vi "log in.vi"() -> ()   [LabVIEW 2016]
uses:
  <vilib>/Utility/config.llb/Read Key (Boolean).vi
  <vilib>/Utility/config.llb/Write Key (String).vi
  <vilib>/Utility/config.llb/Write Key (Boolean).vi
  <vilib>/Utility/config.llb/Read Key (String).vi
  <vilib>/smtpClient/Set Message Text.vi
  <vilib>/Utility/config.llb/NI_LVConfig.lvlib
  <vilib>/smtpClient/LabVIEWSMTPClient.lvlib
panel:
  in  "Sair":bool
  out "error out":errorcluster
  in  "nagevação":enum32{"log in", "cadastrar novo usuário"}(tab)
  in  "Esqueceu a senha":bool
  out "errada":string="Senha ou Usuários incorretos"
  in  "Senha":string
  in  "Usuário":string
  in  "Entrar":bool
  in  "remember":bool
  in  "novo_user":bool
  in  "Voltar":bool
  in  "novamente":string caption="Digite a senha novamente"
  in  "Digite a senha":string
  in  "Usuário":string
  in  "Cadastrar":bool
  # "Cadastrar novo usuário"
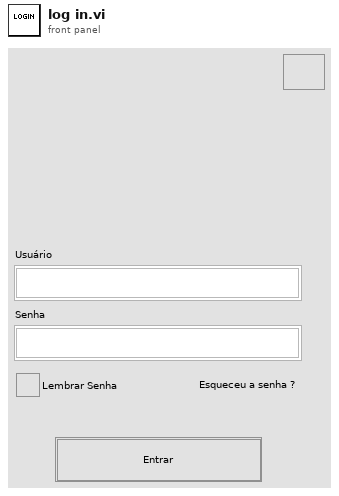
[diagram p1: front panel]
types:
  T1 = typedef "NI_LVConfig.lvlib/Config Data RefNum.ctl" = refnum<k1>
  T2 = typedef "LabVIEWSMTPClient.lvlib/SmtpClientHandle.ctl" = refnum<k1>
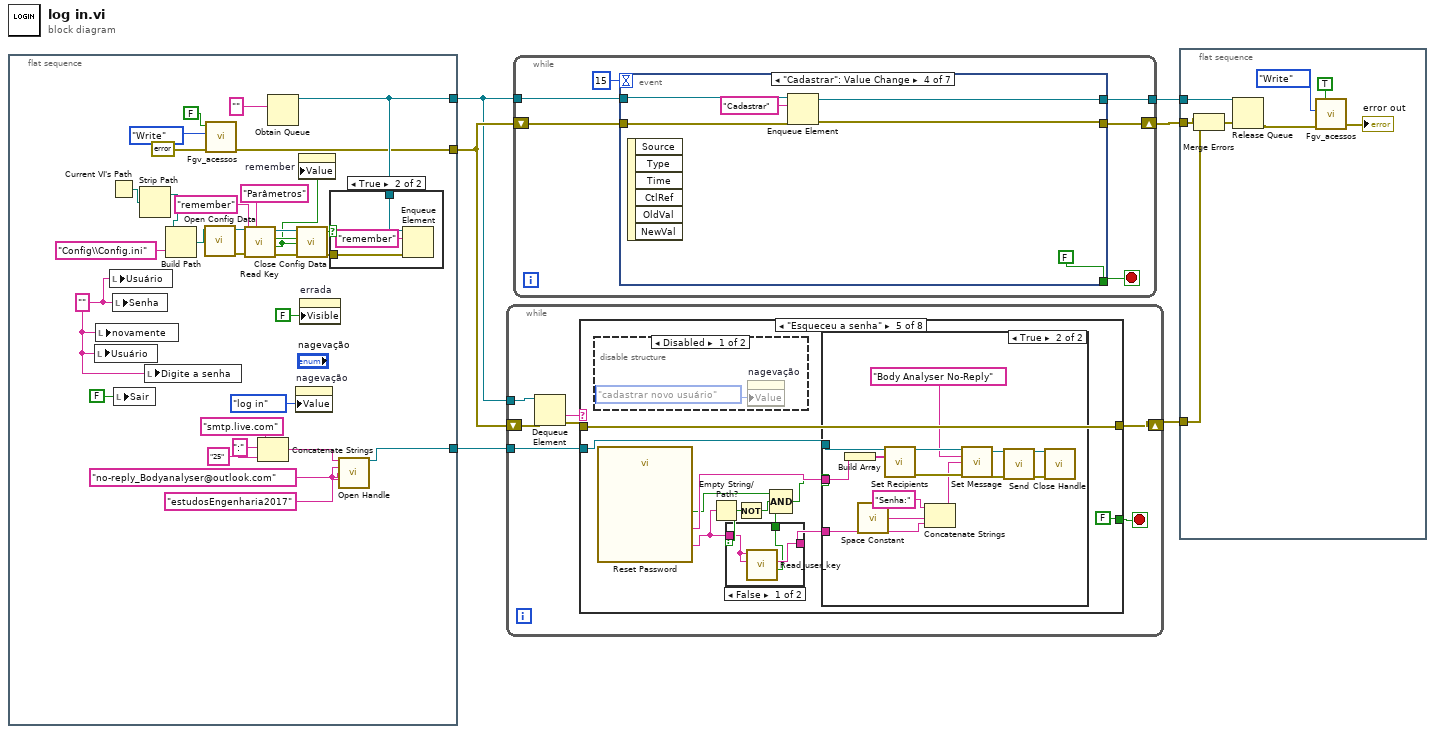
[diagram p0: block diagram]
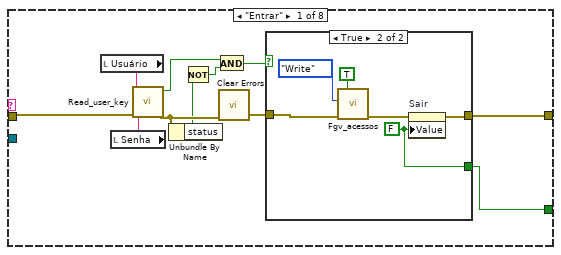
[diagram p2: hidden frame]
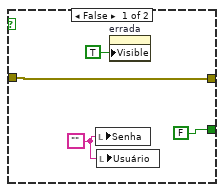
[diagram p3: hidden frame]
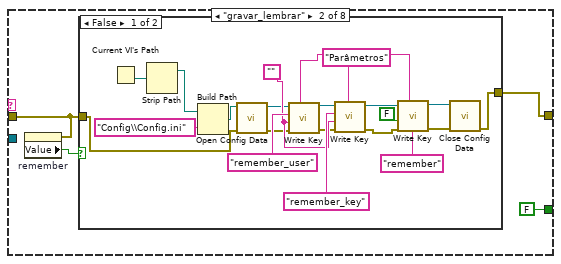
[diagram p4: hidden frame]
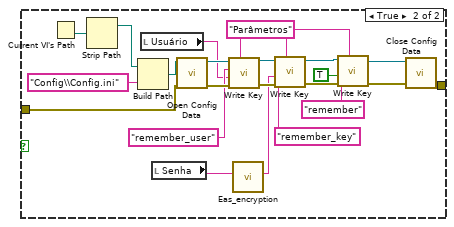
[diagram p5: hidden frame]
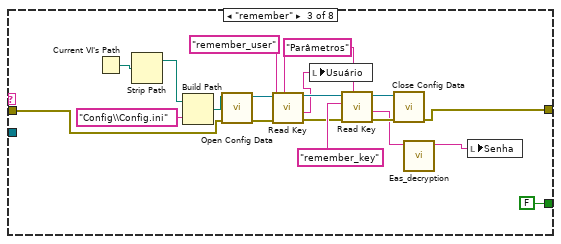
[diagram p6: hidden frame]
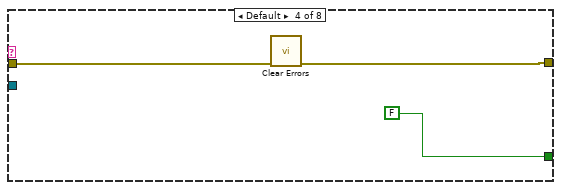
[diagram p7: hidden frame]
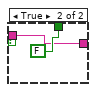
[diagram p8: hidden frame]
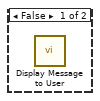
[diagram p9: hidden frame]
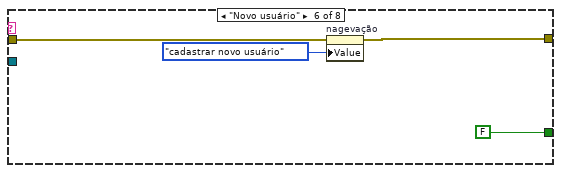
[diagram p11: hidden frame]
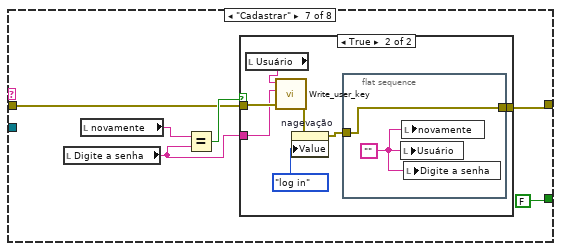
[diagram p12: hidden frame]
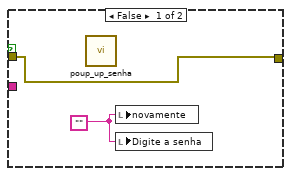
[diagram p13: hidden frame]
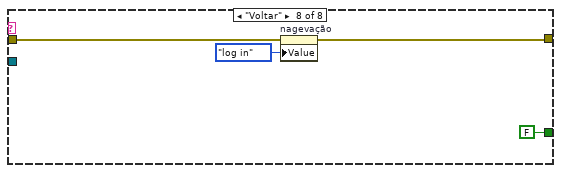
[diagram p14: hidden frame]
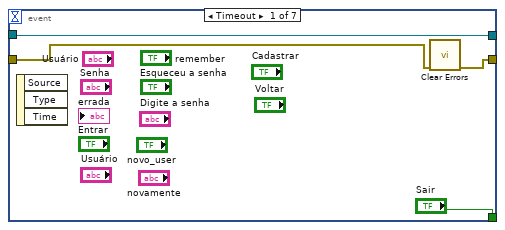
[diagram p15: hidden frame]
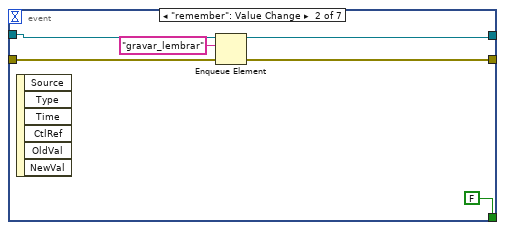
[diagram p16: hidden frame]
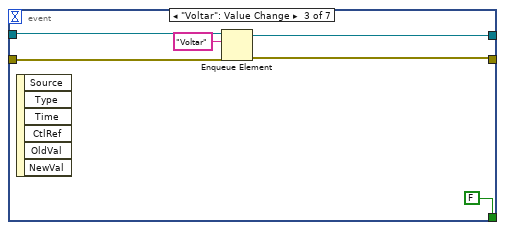
[diagram p17: hidden frame]
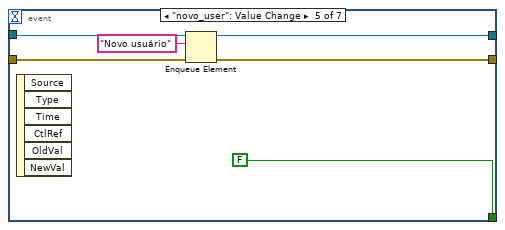
[diagram p18: hidden frame]
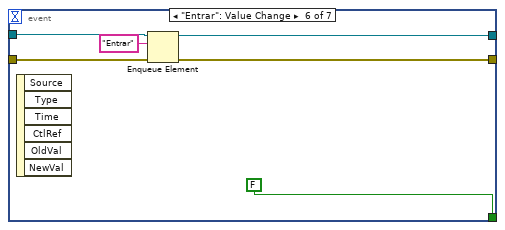
[diagram p19: hidden frame]
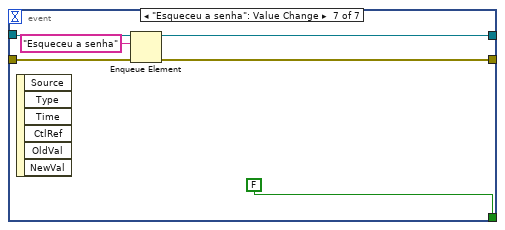
[diagram p20: hidden frame]
diagram:
  n1 = flat-sequence {
    tunnel: [w16] -> w6
    tunnel: [w17] -> w3
    tunnel: [w7] -> w1
    frame #0 {
      w9 = "no-reply_Bodyanalyser@outlook.com" ("from")
      w32 = "" ("Senha")
      n2 = local write "Usuário"(w32) -> ()
      n3 = local write "novamente"(w32) -> ()
      n4 = Current VI's Path() -> (path=w23:path)
      n5 = local write "Usuário"(w32) -> ()
      n6 = local write "Senha"(w32) -> ()
      n7 = local write "Sair"(FALSE ("Sair")) -> ()
      n8 = Strip Path(path=w23) -> (stripped path=w22:path)  [unwired: 1 out]
      n9 = local write "Digite a senha"(w32) -> ()
      n10 = Build Path(base path=w22, name or relative path="Config\\Config.ini") -> (appended path=w20:path)
      n11 = call <vilib>:"Open Config Data.vi"("configuration file path"=w20) -> ("error out"=w28:errorcluster, "refnum"=w27:T1)  [unwired: 8 in, 1 out]
      n12 = call "Fgv_acessos.vi"("error in"=errorcluster {"status"=FALSE, "code"=0, "source"=""} ("error constant"), "Tipo"=enum16{"Write", "Read"}."Write", "Log in _acesso"=FALSE) -> ("Error out"=w16:errorcluster)  [unwired: 7 in, 1 out]
      n13 = call-poly <vilib>:"Read Key.vi"("section"="Parâmetros", "error in (no error)"=w28, "key"="remember", "refnum"=w27) -> ("error out"=w26:errorcluster, "value"=w14:bool, "found?"=w25:bool, "refnum out"=w24:T1)  [unwired: 4 in]
      n14 = Concatenate Strings("smtp.live.com" ("server address"), ":" ("string"), "25" ("string")) -> (w10:string)
      n15 = Obtain Queue(element data type="" ("name (unnamed)")) -> (queue out=w17:refnum<queue>)  [unwired: 4 in, 2 out]
      n16 = property on="nagevação" class="TabCtl (strict)"("Value"=enum32{"log in", "cadastrar novo usuário"}."log in" ("nagevação")) -> ()  [unwired: 2 in, 2 out]
      n17 = call <vilib>:"Close Config Data.vi"("error in (no error)"=w26, "write file if changed (T)"=w25, "refnum"=w24) -> ("error out"=w15:errorcluster)  [unwired: 7 in, 1 out]
      n18 = property on="remember" class="Bool (strict)"("Value"=w14) -> ()  [unwired: 2 in, 2 out]
      n19 = property on="errada" class="Str"("Visible"=FALSE) -> ()  [unwired: 2 in, 2 out]
      n20 = case shown="True" w14 {
        tunnel: w17 -> [_ w39]
        tunnel: w15 -> [_ w38]
        frame False {
        }
        frame True {
          n21 = Enqueue Element(queue=w39, element="remember", error in (no error)=w38) -> ()  [unwired: 1 in, 3 out]
        }
      }
      n22 = call <vilib>:"Open Handle.vi"("server address"=w10, "from"=w9, "username"=w9, "password"="estudosEngenharia2017") -> ("handle out"=w7:T2)  [unwired: 10 in, 1 out]
    }
  }
  n23 = while {
    shift-right: [w44] -> w4
    shift-left: w6 -> [w45]
    tunnel: w3 -> [w42]
    tunnel: w1 -> [w40]
    stop <- w41 stop-if-true
    n24 = Dequeue Element(queue=w42, error in (no error)=w45) -> (element=w46:string, error out=w43:errorcluster)  [unwired: 1 in, 2 out]
    n25 = case shown="\"Esqueceu a senha\"" w46 {
      tunnel: [w53 w70 w118 w133 w146 w169 w172 w189] -> w44
      tunnel: w43 -> [w57 w69 w128 w134 w146 w170 w173 w190]
      tunnel: [w54 FALSE ("Sair") FALSE ("Sair") FALSE FALSE FALSE FALSE FALSE ("Sair")] -> w41
      tunnel: w40 -> [_ _ _ _ w144 _ _ _]
      frame "Entrar" {
        n26 = local read "Usuário"() -> (w56:string)
        n27 = local read "Senha"() -> (w55:string)
        n28 = call "Read_user_key.vi"("Error in"=w57, "Senha"=w55, "User"=w56) -> ("Error out"=w51:errorcluster, "Dados Válidos"=w48:bool)  [unwired: 5 in, 2 out]
        n29 = Unbundle By Name(w51) -> ("status"=w50:bool)
        n30 = Not(x=w50) -> (.not. x?=w49:bool)
        n31 = And(x=w48, y=w49) -> (x .and. y?=w47:bool)
        n32 = call <vilib>:"Clear Errors.vi"("error in (no error)"=w51) -> ("error out"=w52:errorcluster)  [unwired: 5 in, 1 out]
        n33 = case shown="True" w47 {
          tunnel: [FALSE w67] -> w54
          tunnel: w52 -> [w58 w63]
          tunnel: [w58 w66] -> w53
          frame False {
            w60 = ""
            n34 = local write "Senha"(w60) -> ()
            n35 = local write "Usuário"(w60) -> ()
            n36 = property on="errada" class="Str"("Visible"=TRUE) -> ()  [unwired: 2 in, 2 out]
          }
          frame True {
            w67 = FALSE ("Sair")
            n37 = call "Fgv_acessos.vi"("error in"=w63, "Tipo"=enum16{"Write", "Read"}."Write", "Log in _acesso"=TRUE) -> ("Error out"=w62:errorcluster)  [unwired: 7 in, 1 out]
            n38 = property on="Sair" class="Bool (strict)"(error in=w62, "Value"=w67) -> (error out=w66:errorcluster)  [unwired: 1 in, 1 out]
          }
        }
      }
      frame "gravar_lembrar" {
        n39 = property on="remember" class="Bool (strict)"(error in=w69) -> ("Value"=w68:bool)  [unwired: 1 in, 2 out]
        n40 = case shown="False" w68 {
          tunnel: w69 -> [w87 w111]
          tunnel: [w78 w104] -> w70
          frame False {
            w76 = ""
            w86 = "Parâmetros" ("section")
            n41 = Current VI's Path() -> (path=w91:path)
            n42 = Strip Path(path=w91) -> (stripped path=w90:path)  [unwired: 1 out]
            n43 = Build Path(base path=w90, name or relative path="Config\\Config.ini") -> (appended path=w88:path)
            n44 = call <vilib>:"Open Config Data.vi"("error in (no error)"=w87, "configuration file path"=w88) -> ("error out"=w74:errorcluster, "refnum"=w75:T1)  [unwired: 7 in, 1 out]
            n45 = call-poly <vilib>:"Write Key.vi"("section"=w86, "error in (no error)"=w74, "value"=w76, "key"="remember_user", "refnum"=w75) -> ("error out"=w73:errorcluster, "refnum out"=w72:T1)  [unwired: 4 in, 1 out]
            n46 = call-poly <vilib>:"Write Key.vi"("section"=w86, "error in (no error)"=w73, "value"=w76, "key"="remember_key", "refnum"=w72) -> ("error out"=w82:errorcluster, "refnum out"=w81:T1)  [unwired: 4 in, 1 out]
            n47 = call-poly <vilib>:"Write Key.vi"("section"=w86, "error in (no error)"=w82, "value"=FALSE, "key"="remember", "refnum"=w81) -> ("error out"=w79:errorcluster, "refnum out"=w80:T1)  [unwired: 4 in, 1 out]
            n48 = call <vilib>:"Close Config Data.vi"("error in (no error)"=w79, "refnum"=w80) -> ("error out"=w78:errorcluster)  [unwired: 8 in, 1 out]
          }
          frame True {
            w96 = "Parâmetros" ("section")
            n49 = Current VI's Path() -> (path=w113:path)
            n50 = Strip Path(path=w113) -> (stripped path=w112:path)  [unwired: 1 out]
            n51 = Build Path(base path=w112, name or relative path="Config\\Config.ini") -> (appended path=w109:path)
            n52 = local read "Usuário"() -> (w101:string)
            n53 = local read "Senha"() -> (w100:string)
            n54 = call <vilib>:"Open Config Data.vi"("error in (no error)"=w111, "configuration file path"=w109) -> ("error out"=w108:errorcluster, "refnum"=w107:T1)  [unwired: 7 in, 1 out]
            n55 = call-poly <vilib>:"Write Key.vi"("section"=w96, "error in (no error)"=w108, "value"=w101, "key"="remember_user", "refnum"=w107) -> ("error out"=w106:errorcluster, "refnum out"=w105:T1)  [unwired: 4 in, 1 out]
            n56 = call "Eas_encryption.vi"("Key"=w100) -> ("Key"=w99:string)  [unwired: 8 in, 2 out]
            n57 = call-poly <vilib>:"Write Key.vi"("section"=w96, "error in (no error)"=w106, "value"=w99, "key"="remember_key", "refnum"=w105) -> ("error out"=w98:errorcluster, "refnum out"=w97:T1)  [unwired: 4 in, 1 out]
            n58 = call-poly <vilib>:"Write Key.vi"("section"=w96, "error in (no error)"=w98, "value"=TRUE, "key"="remember", "refnum"=w97) -> ("error out"=w93:errorcluster, "refnum out"=w92:T1)  [unwired: 4 in, 1 out]
            n59 = call <vilib>:"Close Config Data.vi"("error in (no error)"=w93, "refnum"=w92) -> ("error out"=w104:errorcluster)  [unwired: 8 in, 1 out]
          }
        }
      }
      frame "remember" {
        w125 = "Parâmetros" ("section")
        n60 = Current VI's Path() -> (path=w132:path)
        n61 = Strip Path(path=w132) -> (stripped path=w131:path)  [unwired: 1 out]
        n62 = Build Path(base path=w131, name or relative path="Config\\Config.ini") -> (appended path=w129:path)
        n63 = call <vilib>:"Open Config Data.vi"("error in (no error)"=w128, "configuration file path"=w129) -> ("error out"=w127:errorcluster, "refnum"=w126:T1)  [unwired: 7 in, 1 out]
        n64 = call-poly <vilib>:"Read Key.vi"("section"=w125, "error in (no error)"=w127, "key"="remember_user", "refnum"=w126) -> ("error out"=w119:errorcluster, "value"=w116:string, "refnum out"=w124:T1)  [unwired: 4 in, 1 out]
        n65 = local write "Usuário"(w116) -> ()
        n66 = call-poly <vilib>:"Read Key.vi"("section"=w125, "error in (no error)"=w119, "key"="remember_key", "refnum"=w124) -> ("error out"=w120:errorcluster, "value"=w115:string, "refnum out"=w121:T1)  [unwired: 4 in, 1 out]
        n67 = call <vilib>:"Close Config Data.vi"("error in (no error)"=w120, "refnum"=w121) -> ("error out"=w118:errorcluster)  [unwired: 8 in, 1 out]
        n68 = call "Eas_decryption.vi"("Key"=w115) -> ("Key"=w114:string)  [unwired: 9 in, 1 out]
        n69 = local write "Senha"(w114) -> ()
      }
      frame Default {
        n70 = call <vilib>:"Clear Errors.vi"("error in (no error)"=w134) -> ("error out"=w133:errorcluster)  [unwired: 5 in, 1 out]
      }
      frame "Esqueceu a senha" {
        n71 = disable-structure shown="Disabled" {
          frame Disabled {
            n72 = property on="nagevação" class="TabCtl (strict)"("Value"=enum32{"log in", "cadastrar novo usuário"}."cadastrar novo usuário" ("nagevação")) -> ()  [unwired: 2 in, 2 out]
          }
          frame Enabled {
          }
        }
        n73 = call "Reset Password"() -> ("Úsuário"=w137:string, "E-mail"=w143:string, "OK"=w141:bool)  [unwired: 16 in, 1 out]
        n74 = Empty String/Path?(string/path=w137) -> (empty?=w136:bool)
        n75 = case shown="False" w136 {
          tunnel: [w149 w150] -> w142
          tunnel: [w148 FALSE] -> w139
          tunnel: w137 -> [w147 w150]
          frame False {
            n76 = call "Read_user_key.vi"("Senha"=w147, "User"=w147) -> ("x = y?"=w148:bool, "Key"=w149:string)  [unwired: 6 in, 2 out]
          }
          frame True {
          }
        }
        n77 = Not(x=w136) -> (.not. x?=w140:bool)
        n78 = Compound Arithmetic op=AND(w141, w140, w139) -> (w138:bool)
        n79 = case shown="True" w138 {
          tunnel: w144 -> [_ w161]
          tunnel: w143 -> [_ w160]
          tunnel: w142 -> [_ w156]
          frame False {
            n80 = call "Display Message to User"() -> ()  [unwired: 10 in, 2 out]
          }
          frame True {
            n81 = Build Array(w160) -> (w159:string[])
            n82 = call <vilib>:"Space Constant.vi"() -> ("String"=w155:string)
            n83 = call <vilib>:"Set Recipients.vi"("handle in"=w161, "to"=w159) -> ("handle out"=w165:T2, "error out"=w164:errorcluster)  [unwired: 12 in]
            n84 = Concatenate Strings("Senha:" ("plain text message"), w155, w156) -> (w154:string)
            n85 = call-poly <vilib>:"Set Message.vi"("handle in"=w165, "subject"="Body Analyser No-Reply", "plain text message"=w154, "error in (no error)"=w164) -> ("handle out"=w162:T2, "error out"=w163:errorcluster)  [unwired: 10 in]
            n86 = call <vilib>:"Send.vi"("handle in"=w162, "error in (no error)"=w163) -> ("handle out"=w152:T2, "error out"=w153:errorcluster)  [unwired: 11 in, 1 out]
            n87 = call <vilib>:"Close Handle.vi"("handle in"=w152, "error in (no error)"=w153) -> ()  [unwired: 12 in, 2 out]
          }
        }
      }
      frame "Novo usuário" {
        n88 = property on="nagevação" class="TabCtl (strict)"(error in=w170, "Value"=enum32{"log in", "cadastrar novo usuário"}."cadastrar novo usuário" ("nagevação")) -> (error out=w169:errorcluster)  [unwired: 1 in, 1 out]
      }
      frame "Cadastrar" {
        n89 = local read "Digite a senha"() -> (w171:string)
        n90 = local read "novamente"() -> (w175:string)
        n91 = Equal?(x=w175, y=w171) -> (x = y?=w174:bool)
        n92 = case shown="True" w174 {
          tunnel: w173 -> [w178 w185]
          tunnel: [w178 w179] -> w172
          tunnel: w171 -> [_ w183]
          frame False {
            w177 = ""
            n93 = call "poup_up_senha.vi"() -> ()  [unwired: 12 in]
            n94 = local write "novamente"(w177) -> ()
            n95 = local write "Digite a senha"(w177) -> ()
          }
          frame True {
            n96 = local read "Usuário"() -> (w184:string)
            n97 = call "Write_user_key.vi"("Error in"=w185, "Key"=w183, "User"=w184) -> ("error out"=w181:errorcluster)  [unwired: 8 in]
            n98 = property on="nagevação" class="TabCtl (strict)"(error in=w181, "Value"=enum32{"log in", "cadastrar novo usuário"}."log in" ("nagevação")) -> (error out=w180:errorcluster)  [unwired: 1 in, 1 out]
            n99 = flat-sequence {
              tunnel: w180 -> [w187]
              tunnel: [w187] -> w179
              frame #0 {
                w186 = ""
                n100 = local write "Usuário"(w186) -> ()
                n101 = local write "novamente"(w186) -> ()
                n102 = local write "Digite a senha"(w186) -> ()
              }
            }
          }
        }
      }
      frame "Voltar" {
        n103 = property on="nagevação" class="TabCtl (strict)"(error in=w190, "Value"=enum32{"log in", "cadastrar novo usuário"}."log in" ("nagevação")) -> (error out=w189:errorcluster)  [unwired: 1 in, 1 out]
      }
    }
  }
  n104 = while {
    tunnel: w3 -> [w197]
    shift-right: [w195] -> w5
    shift-left: w6 -> [w196]
    tunnel: [w194] -> w2
    stop <- w192 stop-if-true
    n105 = event shown="[3] \"Cadastrar\": Value Change" {
      selector: _ -> [_ _ _ _ _ _ _]
      dyn-events: _ -> [_ _ _ _ _ _ _]
      timeout: 15 -> [_ _ _ _ _ _ _]
      tunnel: w197 -> [w201 w206 w213 w219 w225 w231 w237]
      tunnel: w196 -> [w198 w207 w212 w218 w224 w229 w236]
      tunnel: [w199 w204 w211 w217 w223 w228 w235] -> w195
      tunnel: [w201 w205 w210 w216 w222 w227 w233] -> w194
      tunnel: ["Sair" FALSE ("Sair") FALSE ("Sair") FALSE FALSE FALSE FALSE] -> w192
      event Timeout {
        n106 = event-data() -> ()  [unwired: 1 in, 3 out]
        n107 = call <vilib>:"Clear Errors.vi"("error in (no error)"=w198) -> ("error out"=w199:errorcluster)  [unwired: 5 in, 1 out]
      }
      event "remember": Value Change {
        n108 = event-data() -> ()  [unwired: 1 in, 6 out]
        n109 = Enqueue Element(queue=w206, element="gravar_lembrar", error in (no error)=w207) -> (queue out=w205:refnum<queue>, error out=w204:errorcluster)  [unwired: 1 in, 1 out]
      }
      event "Voltar": Value Change {
        n110 = event-data() -> ()  [unwired: 1 in, 6 out]
        n111 = Enqueue Element(queue=w213, element="Voltar", error in (no error)=w212) -> (queue out=w210:refnum<queue>, error out=w211:errorcluster)  [unwired: 1 in, 1 out]
      }
      event "Cadastrar": Value Change {
        n112 = event-data() -> ()  [unwired: 1 in, 6 out]
        n113 = Enqueue Element(queue=w219, element="Cadastrar", error in (no error)=w218) -> (queue out=w216:refnum<queue>, error out=w217:errorcluster)  [unwired: 1 in, 1 out]
      }
      event "novo_user": Value Change {
        n114 = event-data() -> ()  [unwired: 1 in, 6 out]
        n115 = Enqueue Element(queue=w225, element="Novo usuário", error in (no error)=w224) -> (queue out=w222:refnum<queue>, error out=w223:errorcluster)  [unwired: 1 in, 1 out]
      }
      event "Entrar": Value Change {
        n116 = event-data() -> ()  [unwired: 1 in, 6 out]
        n117 = Enqueue Element(queue=w231, element="Entrar", error in (no error)=w229) -> (queue out=w227:refnum<queue>, error out=w228:errorcluster)  [unwired: 1 in, 1 out]
      }
      event "Esqueceu a senha": Value Change {
        n118 = event-data() -> ()  [unwired: 1 in, 6 out]
        n119 = Enqueue Element(queue=w237, element="Esqueceu a senha", error in (no error)=w236) -> (queue out=w233:refnum<queue>, error out=w235:errorcluster)  [unwired: 1 in, 1 out]
      }
    }
  }
  n120 = flat-sequence {
    tunnel: w5 -> [w245]
    tunnel: w4 -> [w244]
    tunnel: w2 -> [w243]
    frame #0 {
      n121 = Merge Errors(w245, w244) -> (w242:errorcluster)
      n122 = Release Queue(queue=w243, error in (no error)=w242) -> (error out=w239:errorcluster)  [unwired: 1 in, 2 out]
      n123 = call "Fgv_acessos.vi"("error in"=w239, "Tipo"=enum16{"Write", "Read"}."Write", "Log in _acesso"=TRUE) -> ("Error out"=→"error out":errorcluster)  [unwired: 7 in, 1 out]
    }
  }
